vi "Read Graph Legend Props.vi"(8 "error in (no error)":errorcluster, 11 "Graph in":refnum<vi>) -> (0 "error out":errorcluster, 2 "Plot Legend Props":T1, 3 "Graph":refnum<vi>)   [LabVIEW 2020, in "VolatusGUIEditorCore.lvlib"]
uses:
  VolatusGUIEditorCore.lvlib
  Plot Legend Props.ctl
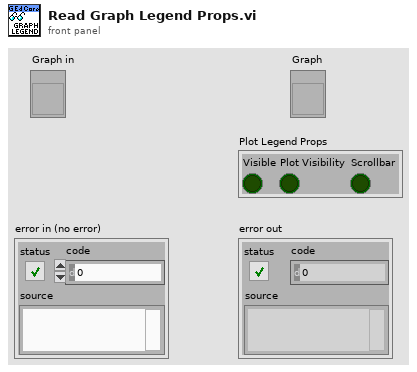
[diagram p1: front panel]
types:
  T1 = typedef "VolatusGUIEditorCore.lvlib/Plot Legend Props.ctl" = cluster{"Visible":bool, "Plot Visibility":bool, "Scrollbar":bool}
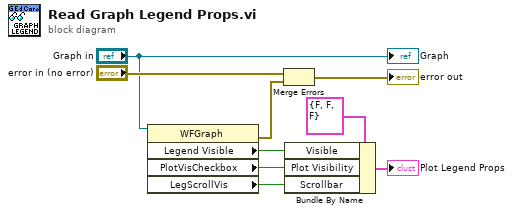
[diagram p0: block diagram]
diagram:
  n1 = property class="WFGraph"(reference="Graph in") -> (error out=w2:errorcluster, "Legend Visible"=w7:bool, "PlotVisCheckbox"=w6:bool, "LegScrollVis"=w5:bool)  [unwired: 1 in, 1 out]
  n2 = Merge Errors("error in (no error)", w2) -> (→"error out":errorcluster)
  n3 = Bundle By Name(cluster=T1 {"Visible"=FALSE, "Plot Visibility"=FALSE, "Scrollbar"=FALSE} ("Plot Legend Props"), "Visible"=w7, "Plot Visibility"=w6, "Scrollbar"=w5) -> (→"Plot Legend Props":T1)
  "Graph" <- "Graph in"
